vi "Read Test Data.vi"(8 "error in":errorcluster, 10 "Sections":u32, 11 "refnum":T2) -> (0 "error out":errorcluster, 2 "Array of tests":T1[](array[typedef]) {"Measurement Res." format="%.0f MHz"; "Blocking Signal" format="%#_gdBm"; "Wanted Signal" format="%#_gdBm"; "Upper Frequency" format="%.0f MHz"; "Lower Frequency" format="%.0f MHz"}, 3 "refnum out":T2)   [LabVIEW 2013]
doc: "This VI will read the test parameters from an ini file into an arrays"
uses:
  <vilib>/Utility/config.llb/Config Data RefNum.ctl
  Master Test Parameters.ctl
  <vilib>/Utility/config.llb/Read Key (U32).vi
  <vilib>/Utility/config.llb/Read Key (Double).vi
  <vilib>/Utility/config.llb/NI_LVConfig.lvlib
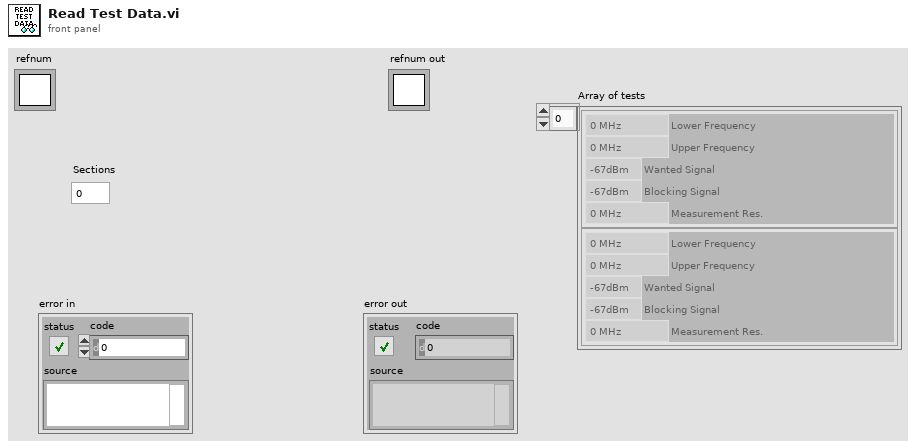
[diagram p1: front panel]
types:
  T1 = typedef "Master Test Parameters.ctl" = cluster{"Lower Frequency":u32, "Upper Frequency":u32, "Wanted Signal":dbl, "Blocking Signal":dbl, "Measurement Res.":u32}
  T2 = typedef "NI_LVConfig.lvlib/Config Data RefNum.ctl" = refnum<k1>
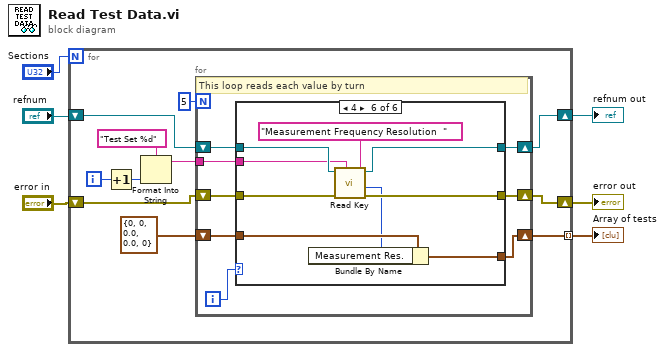
[diagram p0: block diagram]
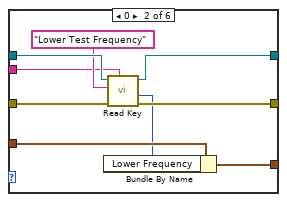
[diagram p3: hidden frame]
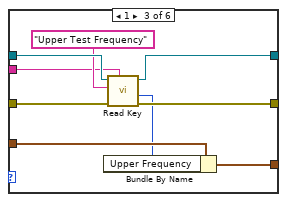
[diagram p4: hidden frame]
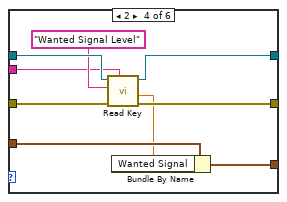
[diagram p5: hidden frame]
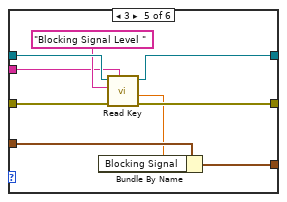
[diagram p6: hidden frame]
diagram:
  n1 = for {
    N: "Sections" -> [_]
    shift-right: [w10] -> w4
    shift-left: "refnum" -> [w11]
    tunnel: [w9] -> w3 mode=indexing
    shift-right: [w8] -> w1
    shift-left: "error in" -> [w7]
    i -> [w16]
    n2 = Increment(x=w16) -> (x+1=w15:i32)
    n3 = Format Into String(format string="Test Set %d", w15) -> (resulting string=w12:string)  [unwired: 2 in, 1 out]
    n4 = for {
      N: 5 -> [_]
      shift-right: [w24] -> w10
      shift-left: w11 -> [w23]
      shift-right: [w22] -> w9
      shift-left: T1 {"Lower Frequency"=0, "Upper Frequency"=0, "Wanted Signal"=0.0, "Blocking Signal"=0.0, "Measurement Res."=0} ("element") -> [w21]
      shift-right: [w20] -> w8
      shift-left: w7 -> [w19]
      tunnel: w12 -> [w18]
      i -> [w25]
      # "This loop reads each value by turn"
      n5 = case shown="4" w25 {
        tunnel: [w27 w37 w46 w55 w64 w73] -> w24
        tunnel: w23 -> [w27 w36 w45 w54 w63 w72]
        tunnel: [w28 w34 w43 w52 w61 w70] -> w22
        tunnel: w21 -> [w28 w33 w42 w51 w60 w69]
        tunnel: [w26 w32 w41 w50 w59 w68] -> w20
        tunnel: w19 -> [w26 w31 w40 w49 w58 w67]
        tunnel: w18 -> [_ w30 w39 w48 w57 w66]
        frame Default {
        }
        frame 0 {
          n6 = call-poly <vilib>:"Read Key.vi"("section"=w30, "error in (no error)"=w31, "key"="Lower Test Frequency", "refnum"=w36) -> ("error out"=w32:errorcluster, "value"=w29:u32, "refnum out"=w37:T2)  [unwired: 4 in, 1 out]
          n7 = Bundle By Name(cluster=w33, "Lower Frequency"=w29) -> (w34:T1)
        }
        frame 1 {
          n8 = call-poly <vilib>:"Read Key.vi"("section"=w39, "error in (no error)"=w40, "key"="Upper Test Frequency", "refnum"=w45) -> ("error out"=w41:errorcluster, "value"=w38:u32, "refnum out"=w46:T2)  [unwired: 4 in, 1 out]
          n9 = Bundle By Name(cluster=w42, "Upper Frequency"=w38) -> (w43:T1)
        }
        frame 2 {
          n10 = call-poly <vilib>:"Read Key.vi"("section"=w48, "error in (no error)"=w49, "key"="Wanted Signal Level", "refnum"=w54) -> ("error out"=w50:errorcluster, "value"=w47:dbl, "refnum out"=w55:T2)  [unwired: 4 in, 1 out]
          n11 = Bundle By Name(cluster=w51, "Wanted Signal"=w47) -> (w52:T1)
        }
        frame 3 {
          n12 = call-poly <vilib>:"Read Key.vi"("section"=w57, "error in (no error)"=w58, "key"="Blocking Signal Level ", "refnum"=w63) -> ("error out"=w59:errorcluster, "value"=w56:dbl, "refnum out"=w64:T2)  [unwired: 4 in, 1 out]
          n13 = Bundle By Name(cluster=w60, "Blocking Signal"=w56) -> (w61:T1)
        }
        frame 4 {
          n14 = call-poly <vilib>:"Read Key.vi"("section"=w66, "error in (no error)"=w67, "key"="Measurement Frequency Resolution  ", "refnum"=w72) -> ("error out"=w68:errorcluster, "value"=w65:u32, "refnum out"=w73:T2)  [unwired: 4 in, 1 out]
          n15 = Bundle By Name(cluster=w69, "Measurement Res."=w65) -> (w70:T1)
        }
      }
    }
  }
  "refnum out" <- w4
  "Array of tests" <- w3
  "error out" <- w1
